vi "DigitalPulseTrain.vi"() -> ()   [LabVIEW 2017]
uses:
  <vilib>/DAQmx/create/channels.llb/DAQmx Create Channel (CO-Pulse Generation-Frequency).vi
  <vilib>/DAQmx/configure/timing.llb/DAQmx Timing (Implicit).vi
  <resource>/objmgr/daqmx.rc
panel:
  out "CO.Pulse.DutyCyc":dbl
  out "CO.Pulse.Freq":dbl
  in  "Channel Settings":T1={"Frequency"=10.0, "Duty Cycle"=0.5, "counter"="Dev6/ctr0", "Output Terminal"="/Dev6/PFI12"} {"Duty Cycle" min=0.01 max=0.99 format="%_6g"; "Frequency" min=1.0 max=1000000.0 format="%_6f"}
  in  "stop":bool
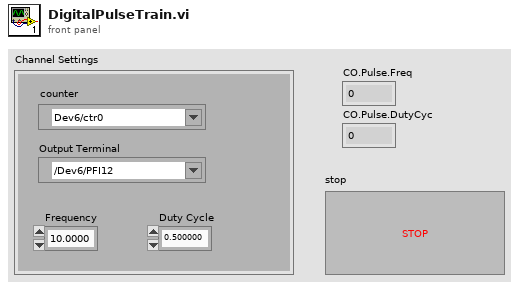
[diagram p1: front panel]
types:
  T1 = cluster{"Frequency":dbl, "Duty Cycle":dbl, "counter":tag, "Output Terminal":tag}
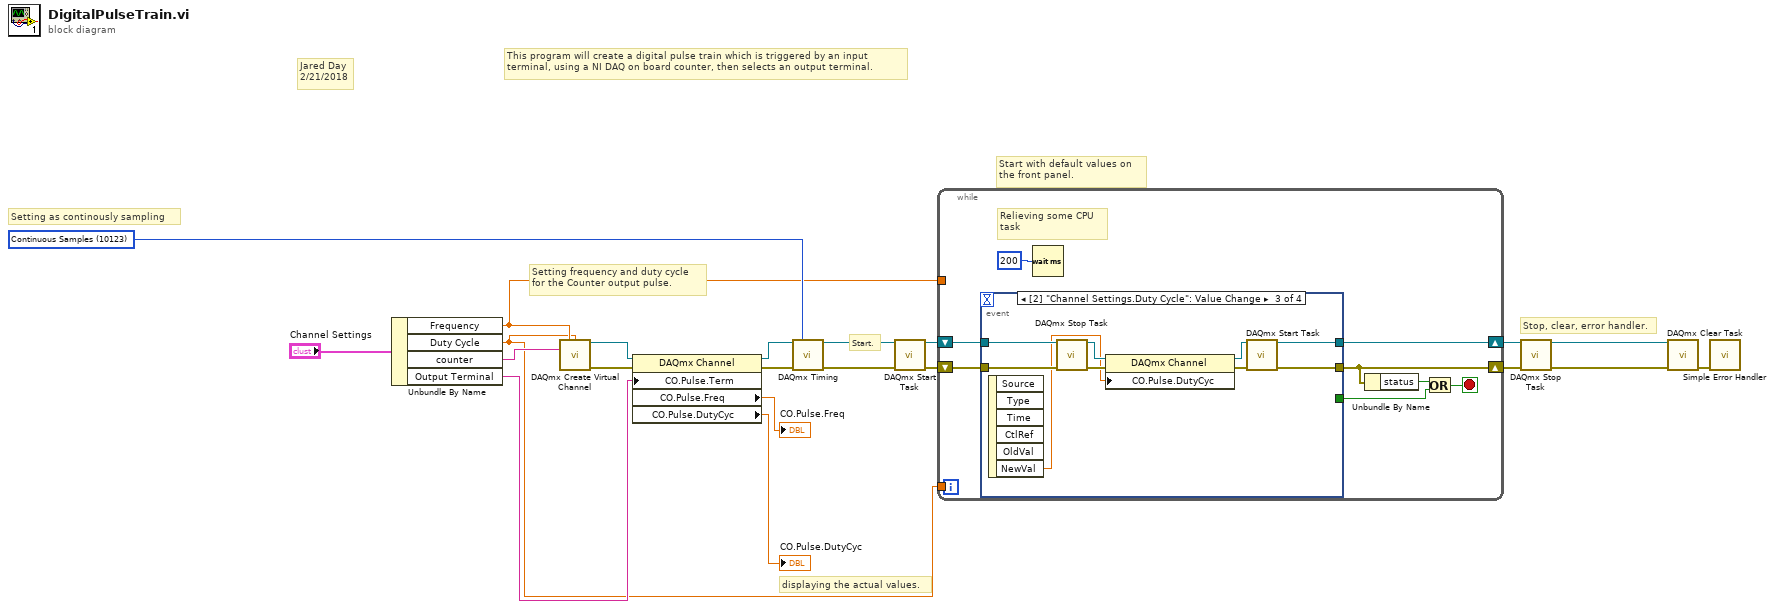
[diagram p0: block diagram]
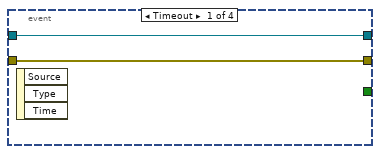
[diagram p2: hidden frame]
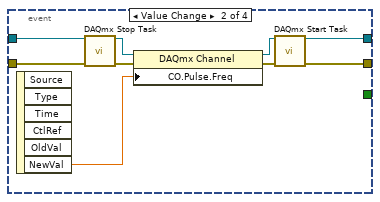
[diagram p3: hidden frame]
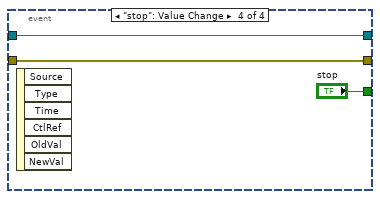
[diagram p4: hidden frame]
diagram:
  w9 = 10123 items=["Finite Samples"=10178, "Continuous Samples"=10123, "Hardware Timed Single Point"=12522] ("sample mode")
  # "Setting as continously sampling"
  # "displaying the actual values."
  # "Setting frequency and duty cycle\nfor the Counter output pulse."
  # "Start."
  # "Start with default values on \nthe front panel."
  # "Stop, clear, error handler."
  # "This program will create a digital pulse train which is triggered by an input\nterminal, using a NI DAQ on board counter, then selects an output terminal."
  # "Jared Day\n2/21/2018"
  n1 = Unbundle By Name("Channel Settings") -> ("Frequency"=w4:dbl, "Duty Cycle"=w3:dbl, "counter"=w16:tag, "Output Terminal"=w8:tag)
  n2 = call-poly <vilib>:"DAQmx Create Virtual Channel.vi"("frequency"=w4, "duty cycle"=w3, "counter"=w16) -> ("task out"=w13:refnum<k21>, "error out"=w12:errorcluster)  [unwired: 11 in]
  n3 = property class="DAQmx Channel"(reference=w13, error in=w12, "CO.Pulse.Term"=w8) -> (reference out=w11:refnum<k21>, error out=w10:errorcluster, "CO.Pulse.Freq"=→"CO.Pulse.Freq":dbl, "CO.Pulse.DutyCyc"=→"CO.Pulse.DutyCyc":dbl)
  n4 = call-poly <vilib>:"DAQmx Timing.vi"("task/channels in"=w11, "sample mode"=w9, "error in"=w10) -> ("task out"=w2:refnum<k21>, "error out"=w1:errorcluster)  [unwired: 11 in]
  n5 = call <vilib>:"DAQmx Start Task.vi"("task/channels in"=w2, "error in"=w1) -> ("task out"=w6:refnum<k21>, "error out"=w5:errorcluster)  [unwired: 12 in]
  n6 = while {
    shift-right: [w25] -> w21
    shift-left: w6 -> [w27]
    shift-right: [w24] -> w20
    shift-left: w5 -> [w26]
    tunnel: w4 -> [_]
    tunnel: w3 -> [_]
    stop <- w29 stop-if-true
    # "Relieving some CPU\ntask"
    n7 = event shown="[2] \"Channel Settings.Duty Cycle\": Value Change" {
      selector: _ -> [_ _ _ _]
      dyn-events: _ -> [_ _ _ _]
      timeout: _ -> [_ _ _ _]
      tunnel: w27 -> [w31 w40 w49 w51]
      tunnel: w26 -> [w30 w39 w48 w50]
      tunnel: [w31 w36 w43 w51] -> w25
      tunnel: [w30 w35 w42 w50] -> w24
      tunnel: [_ _ _ "stop"] -> w22
      event Timeout {
        n8 = event-data() -> ()  [unwired: 1 in, 3 out]
      }
      event "Channel Settings.Frequency": Value Change {
        n9 = event-data() -> ("NewVal"=w32:dbl)  [unwired: 1 in, 5 out]
        n10 = call <vilib>:"DAQmx Stop Task.vi"("task/channels in"=w40, "error in"=w39) -> ("task out"=w38:refnum<k21>, "error out"=w37:errorcluster)  [unwired: 12 in]
        n11 = property class="DAQmx Channel"(reference=w38, error in=w37, "CO.Pulse.Freq"=w32) -> (reference out=w34:refnum<k21>, error out=w33:errorcluster)
        n12 = call <vilib>:"DAQmx Start Task.vi"("task/channels in"=w34, "error in"=w33) -> ("task out"=w36:refnum<k21>, "error out"=w35:errorcluster)  [unwired: 12 in]
      }
      event "Channel Settings.Duty Cycle": Value Change {
        n13 = event-data() -> ("NewVal"=w41:dbl)  [unwired: 1 in, 5 out]
        n14 = call <vilib>:"DAQmx Stop Task.vi"("task/channels in"=w49, "error in"=w48) -> ("task out"=w47:refnum<k21>, "error out"=w46:errorcluster)  [unwired: 12 in]
        n15 = property class="DAQmx Channel"(reference=w47, error in=w46, "CO.Pulse.DutyCyc"=w41) -> (reference out=w45:refnum<k21>, error out=w44:errorcluster)
        n16 = call <vilib>:"DAQmx Start Task.vi"("task/channels in"=w45, "error in"=w44) -> ("task out"=w43:refnum<k21>, "error out"=w42:errorcluster)  [unwired: 12 in]
      }
      event "stop": Value Change {
        n17 = event-data() -> ()  [unwired: 1 in, 6 out]
      }
    }
    n18 = Wait (ms)(milliseconds to wait=200) -> ()  [unwired: 1 out]
    n19 = Unbundle By Name(w24) -> ("status"=w23:bool)
    n20 = Or(x=w23, y=w22) -> (x .or. y?=w29:bool)
  }
  n21 = call <vilib>:"DAQmx Stop Task.vi"("task/channels in"=w21, "error in"=w20) -> ("task out"=w19:refnum<k21>, "error out"=w18:errorcluster)  [unwired: 12 in]
  n22 = call <vilib>:"DAQmx Clear Task.vi"("task in"=w19, "error in"=w18) -> ("error out"=w17:errorcluster)  [unwired: 13 in]
  n23 = call <vilib>:"Simple Error Handler.vi"("error in (no error)"=w17) -> ()  [unwired: 4 in, 5 out]
